vi "FIR Filter with I.C..vi"   [LabVIEW 2024, in "NI_AALBase.lvlib"]
doc: "<p>Filters the input sequence <strong>X</strong> using the direct-form FIR filter specified by <strong>FIR Coefficients</strong>. You can use this VI to process blocks of continuous data. Wire data to the <strong>X</strong> input to determine the polymorphic instance to use or <a href=\"nihelplauncher://docs/csh?context=lvcore_lvhowto_selectingdefaultinstpolyvi\">manually select</a> the instance.</p>"
uses:
  NI_AALBase.lvlib
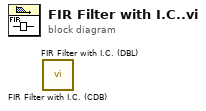
[diagram p0: block diagram]
diagram:
  n1 = call "FIR Filter with I.C. (CDB).vi"() -> ()  [unwired: 8 in, 3 out]
  n2 = call "FIR Filter with I.C. (DBL).vi"() -> ()  [unwired: 8 in, 3 out]
